vi "Allocate Calculation Batch.vi"(0 "GPU FFT Calculator in":refnum<class "GPU FFT Calculator.lvclass">, 1 "Amount of Batches":i32, 2 "Batch Index":i32, 5 "Download DMA Manager":refnum<class "DMA Manager.lvclass">, 7 "Upload DMA Manager":refnum<class "DMA Manager.lvclass">, 9 "Dataset":i16[](array[numeric]), 11 "error in (no error)":errorcluster, 12 "Frame Size":u64, 13 "Data Offset In":u64) -> (4 "Data Offset Out":u64, 6 "Calculation Batch":T1 {"Zoom Parameters"."fwidth:" format="%#_6p"; "Zoom Parameters"."f0:" format="%#_6p"}, 15 "error out":errorcluster)   [LabVIEW 2020, in "GPU FFT Calculator.lvlib" / "GPU FFT Calculator.lvclass"]
uses:
  GPU FFT Calculator/GPU FFT Calculator/GPU FFT Calculator.lvclass
  <vilib>/Natan Biesmans/G2CPU GPU and CPU HPC Toolkit/G2CPU Libraries/Async IO/DMA Manager/DMA Manager.lvclass
  C:/Users/natan/Documents/G2CPU-Performance-Demo/Calculation Worker/Calculation Worker/Calculation Worker.lvclass
  GPU FFT Calculator/GPU FFT Calculator/GPU Calculation Message.ctl
  <vilib>/Natan Biesmans/G2CPU GPU and CPU HPC Toolkit/G2CPU Libraries/Arrays/1DArray/s16/1D Array s16.lvclass
  C:/Program Files/National Instruments/LabVIEW 2026/vi.lib/Natan Biesmans/G2CPU GPU and CPU HPC Toolkit/G2CPU Libraries/Arrays/Array/Array Prototype.lvclass
  <vilib>/Natan Biesmans/G2CPU GPU and CPU HPC Toolkit/G2CPU Libraries/Arrays/1DArray/f32/1D Array f32.lvclass
  chart zoom.ctl
  GPU FFT Calculator/GPU FFT Calculator/GPU Metrics.ctl
  GPU FFT Calculator/GPU FFT Calculator/GPU FFT Calculator.lvclass/GPU FFT Calculator.ctl
  cdea0ef2-3c0b-4c71-89d1-4dccbf828d85.vi
  b71bdd0b-bcfd-4d30-a3ca-9e0d31e18c76.vi
  cdea0ef2-3c0b-4c71-89d1-4dccbf828d85.vi/c1c6ba82-99b7-4273-a704-85eea64f3b4b.vi
  <vilib>/Natan Biesmans/G2CPU GPU and CPU HPC Toolkit/G2CPU Libraries/Arrays/SubVI/Handle CUDA Error.vi
  cdea0ef2-3c0b-4c71-89d1-4dccbf828d85.vi/fcfd33d5-6ac1-42cc-9267-61f2760a5aae.vi
  <vilib>/Natan Biesmans/G2CPU GPU and CPU HPC Toolkit/ArrayFire Driver/VIs/Run as Multi Device.vi
  cdea0ef2-3c0b-4c71-89d1-4dccbf828d85.vi/8aa0c4af-4daa-4014-9a01-595272b02124.vi
  cdea0ef2-3c0b-4c71-89d1-4dccbf828d85.vi/6d883df8-3b64-4008-8da1-8b1f8b11b48b.vi
  <vilib>/Natan Biesmans/G2CPU GPU and CPU HPC Toolkit/G2CPU Libraries/Runtime Licensing/G2CPU License Check.vi
  b71bdd0b-bcfd-4d30-a3ca-9e0d31e18c76.vi/c1c6ba82-99b7-4273-a704-85eea64f3b4b.vi
  b71bdd0b-bcfd-4d30-a3ca-9e0d31e18c76.vi/fcfd33d5-6ac1-42cc-9267-61f2760a5aae.vi
  b71bdd0b-bcfd-4d30-a3ca-9e0d31e18c76.vi/8aa0c4af-4daa-4014-9a01-595272b02124.vi
  b71bdd0b-bcfd-4d30-a3ca-9e0d31e18c76.vi/6d883df8-3b64-4008-8da1-8b1f8b11b48b.vi
  cdea0ef2-3c0b-4c71-89d1-4dccbf828d85.vi/8aa0c4af-4daa-4014-9a01-595272b02124.vi/c174a7f7-781d-4fed-8bab-bf30bc03dac0.vi
  cdea0ef2-3c0b-4c71-89d1-4dccbf828d85.vi/6d883df8-3b64-4008-8da1-8b1f8b11b48b.vi/313ec8c5-c203-475c-9de0-0583f6fb8b4d.vi
  b71bdd0b-bcfd-4d30-a3ca-9e0d31e18c76.vi/8aa0c4af-4daa-4014-9a01-595272b02124.vi/c174a7f7-781d-4fed-8bab-bf30bc03dac0.vi
  b71bdd0b-bcfd-4d30-a3ca-9e0d31e18c76.vi/6d883df8-3b64-4008-8da1-8b1f8b11b48b.vi/313ec8c5-c203-475c-9de0-0583f6fb8b4d.vi
  <vilib>/Natan Biesmans/G2CPU GPU and CPU HPC Toolkit/G2CPU Libraries/Manage Environment/G2CPU Get Backend.vi
  <vilib>/Utility/error.llb/Error Cluster From Error Code.vi
  <vilib>/Natan Biesmans/G2CPU GPU and CPU HPC Toolkit/G2CPU Libraries/Arrays/SubVI/G2CPU State.vi
  <vilib>/NI License Manager/Open Session.vi
  <vilib>/NI License Manager/Check License Status.vi
  <vilib>/NI License Manager/Check License Status (Single).vi
  <vilib>/NI License Manager/Activate License.vi
  <vilib>/NI License Manager/Activate License (Single).vi
  <vilib>/NI License Manager/Close Session.vi
  <vilib>/Natan Biesmans/G2CPU GPU and CPU HPC Toolkit/ArrayFire Driver/subvi/Error Converter (ErrCode or Status).vi
  <vilib>/Natan Biesmans/G2CPU GPU and CPU HPC Toolkit/G2CPU Libraries/Arrays/Array/G2CPU Set Array Pointer.vi
  <vilib>/Natan Biesmans/G2CPU GPU and CPU HPC Toolkit/ArrayFire Driver/VIs/eval.vi
  <resource>/Natan Biesmans/G2CPU GPU and CPU HPC Toolkit/Garbage Collector/G2CPU DMAGarbageCollectorFGV.vi
  <vilib>/Natan Biesmans/G2CPU GPU and CPU HPC Toolkit/G2CPU Libraries/Arrays/Array/Array Prototype.lvclass
  Simple UI/Simple UI/Simple UI.lvclass
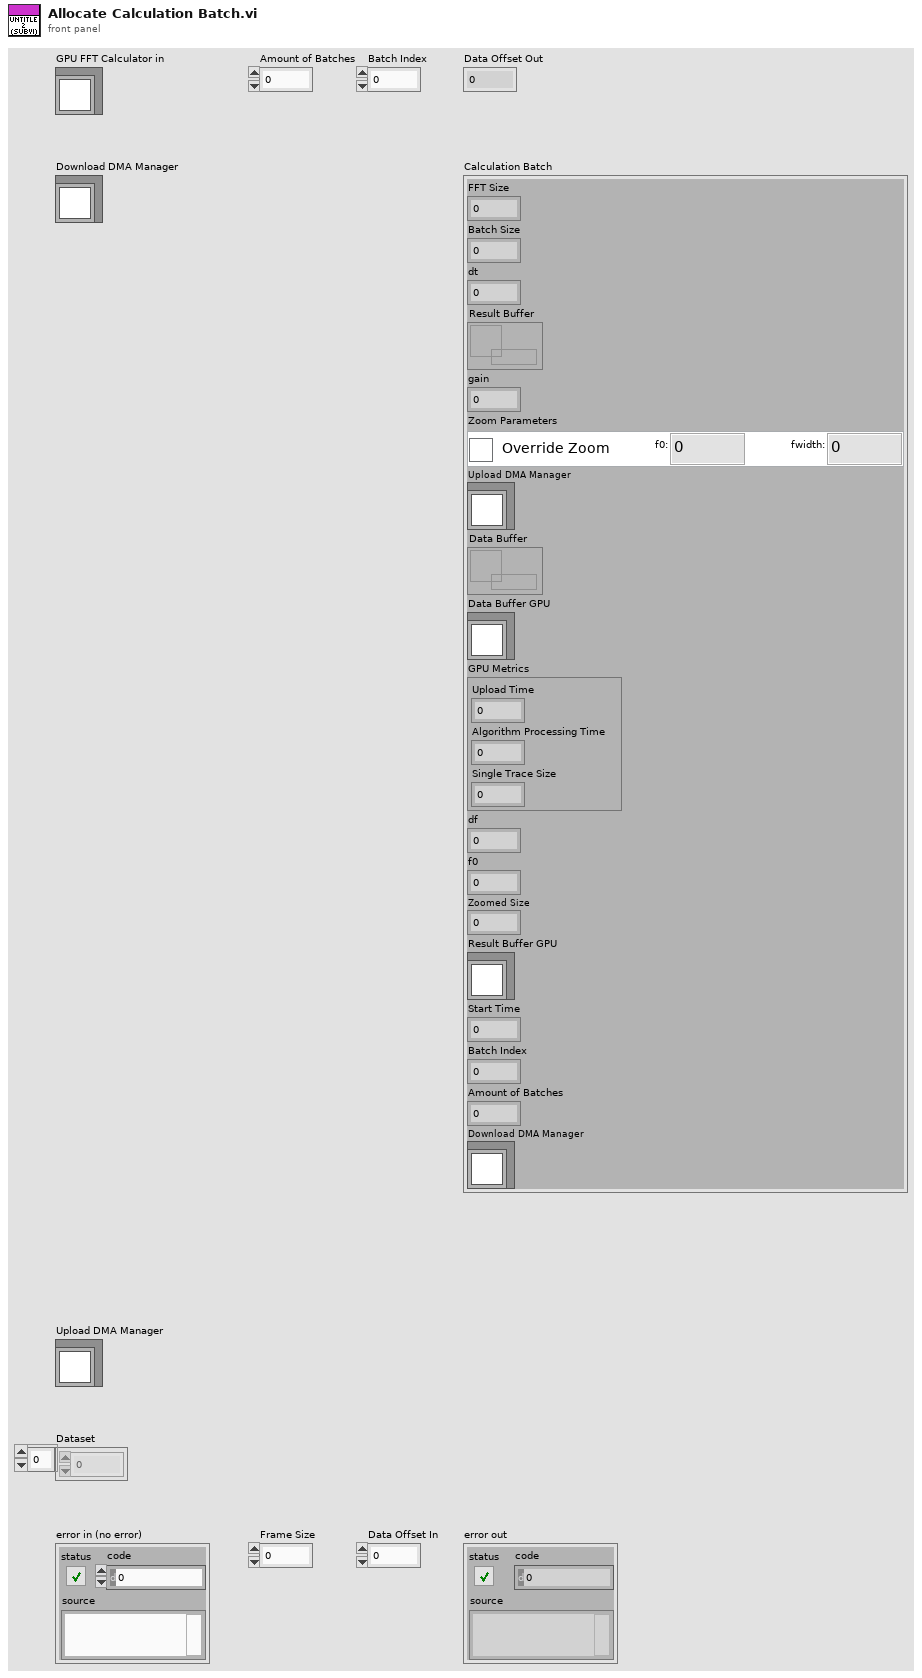
[diagram p1: front panel]
types:
  T1 = typedef "GPU FFT Calculator.lvlib/GPU FFT Calculator.lvclass/GPU Calculation Message.ctl" = cluster{"FFT Size":u64, "Batch Size":u64, "dt":dbl, "Result Buffer":refnum<data-value>, "gain":dbl, "Zoom Parameters":T2, "Upload DMA Manager":refnum<class "DMA Manager.lvclass">, "Data Buffer":refnum<data-value>, "Data Buffer GPU":refnum<class "1D Array s16.lvclass">, "GPU Metrics":T3, "df":dbl, "f0":dbl, "Zoomed Size":u64, "Result Buffer GPU":refnum<class "1D Array f32.lvclass">, "Start Time":dbl, "Batch Index":i32, "Amount of Batches":i32, "Download DMA Manager":refnum<class "DMA Manager.lvclass">}
  T2 = typedef "Simple UI.lvlib/Simple UI.lvclass/chart zoom.ctl" = cluster{"Override":bool, "f0: ":dbl, "fwidth: ":dbl}
  T3 = typedef "GPU FFT Calculator.lvlib/GPU FFT Calculator.lvclass/GPU Metrics.ctl" = cluster{"Upload Time":dbl, "Algorithm Processing Time":dbl, "Single Trace Size":u64}
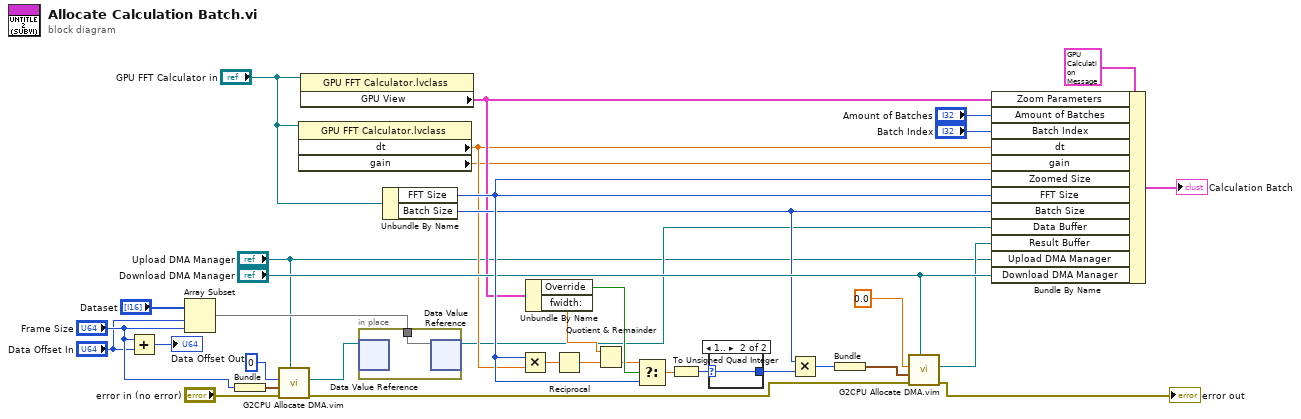
[diagram p0: block diagram]
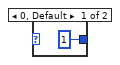
[diagram p2: hidden frame]
diagram:
  n1 = Add(x="Frame Size", y="Data Offset In") -> (x+y=→"Data Offset Out":u64)
  n2 = Array Subset(array="Dataset", index="Data Offset In", length="Frame Size") -> (w9:i16[])
  n3 = Bundle("Frame Size"="Frame Size") -> (w30:cluster{"Frame Size":u64})  [unwired: 1 in]
  n4 = call "G2CPU Allocate DMA.vim"("DMA Manager"="Upload DMA Manager", "error in (no error)"="error in (no error)", "Size"=w30, "Datatype"=i16 0) -> ("error out"=w32:errorcluster, "DMA Memory"=w35:refnum<data-value>)  [unwired: 6 in]
  n5 = property on="Property Node" class="GPU FFT Calculator.lvclass"(reference="GPU FFT Calculator in") -> ("dt"=w18:dbl, "gain"=w11:dbl)  [unwired: 1 in, 2 out]
  n6 = property on="Property Node" class="GPU FFT Calculator.lvclass"(reference="GPU FFT Calculator in") -> ("GPU View"=w19:T2)  [unwired: 1 in, 2 out]
  n7 = in-place "In Place Element Structure" {
    in-place-border: w9 -> [w37]
    n8 = in-place-dvr #1(w35) -> ()  [unwired: 2 out]
    n9 = in-place-dvr #1(w37) -> (w10:refnum<data-value>)  [unwired: 1 out]
  }
  n10 = Unbundle By Name("GPU FFT Calculator in") -> ("FFT Size"=w36:u64, "Batch Size"=w25:u64)
  n11 = Multiply(x=w36, y=w18) -> (x*y=w15:dbl)
  n12 = Unbundle By Name(w19) -> ("Override"=w21:bool, "fwidth:"=w14:dbl)
  n13 = Reciprocal(x=w15) -> (1/x=w16:dbl)
  n14 = Quotient & Remainder(x=w14, y=w16) -> (floor(x/y)=w20:dbl)  [unwired: 1 out]
  n15 = Select(t=w20, s=w21, f=w36) -> (s? t:f=w22:dbl)
  n16 = To Unsigned Quad Integer(1:w22) -> (0:w23:u64)
  n17 = case shown="1.." w23 {
    selector: w23 -> [_ w39]
    tunnel: [u64 1 w39] -> w24
    frame 0, Default {
    }
    frame 1.. {
    }
  }
  n18 = Multiply(x=w25, y=w24) -> (x*y=w1:u64)
  n19 = Bundle(w1) -> (w26:cluster{u64})  [unwired: 1 in]
  n20 = call "G2CPU Allocate DMA.vim"("DMA Manager"="Download DMA Manager", "error in (no error)"=w32, "Size"=w26, "Datatype"=sgl 0.0) -> ("error out"=→"error out":errorcluster, "DMA Memory"=w28:refnum<data-value>)  [unwired: 6 in]
  n21 = Bundle By Name(cluster=T1 {"FFT Size"=0, "Batch Size"=0, "dt"=0.0, "Result Buffer"=refnum, "gain"=0.0, "Zoom Parameters"={"Override"=FALSE, "f0: "=0.0, "fwidth: "=0.0}, "Upload DMA Manager"=refnum, "Data Buffer"=refnum, "Data Buffer GPU"=refnum, "GPU Metrics"={"Upload Time"=0.0, "Algorithm Processing Time"=0.0, "Single Trace Size"=0}, "df"=0.0, "f0"=0.0, "Zoomed Size"=0, "Result Buffer GPU"=refnum, "Start Time"=0.0, "Batch Index"=0, "Amount of Batches"=0, "Download DMA Manager"=refnum} ("element"), "Zoom Parameters"=w19, "Amount of Batches"="Amount of Batches", "Batch Index"="Batch Index", "dt"=w18, "gain"=w11, "Zoomed Size"=w36, "FFT Size"=w36, "Batch Size"=w25, "Data Buffer"=w10, "Result Buffer"=w28, "Upload DMA Manager"="Upload DMA Manager", "Download DMA Manager"="Download DMA Manager") -> (→"Calculation Batch":T1)
